vi "Predet_Inject.vi"   [LabVIEW 2017]
uses:
  <vilib>/DAQmx/write.llb/DAQmx Write (Digital 1D Wfm NChan NSamp).vi
  <vilib>/DAQmx/create/channels.llb/DAQmx Create Channel (DO-Digital Output).vi
  <vilib>/DAQmx/configure/timing.llb/DAQmx Timing (Sample Clock).vi
  <vilib>/Waveform/DWDTOps.llb/DWDT Uncompress Digital.vi
  <vilib>/DAQmx/miscellaneous.llb/DAQmx Fill In Error Info.vi
  <resource>/objmgr/daqmx.rc
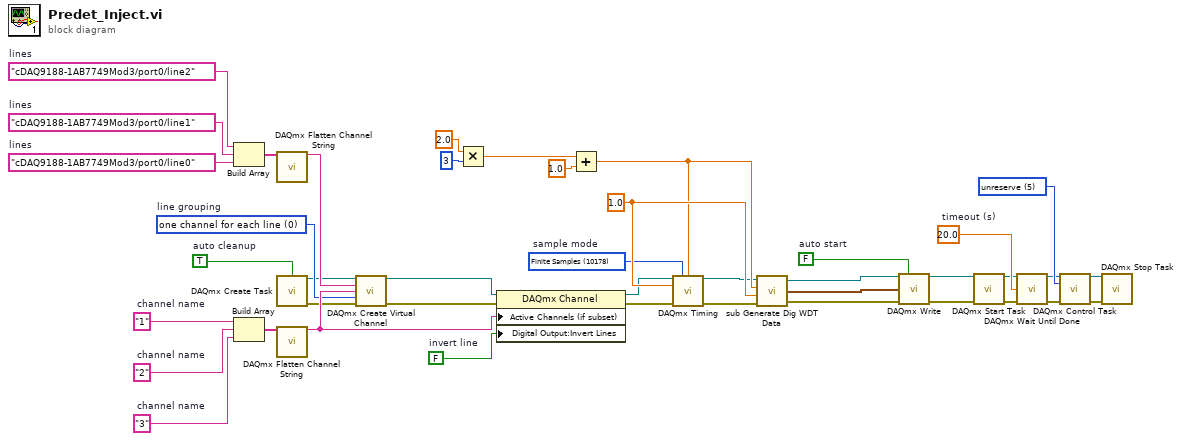
[diagram p0: block diagram]
diagram:
  w42 = 1.0 ("Predet Freq (Hz)")
  w40 = 5 items=["verify"=2, "reserve"=4, "commit"=3, "unreserve"=5, "abort"=6] ("action")
  w31 = "3"  # channel name
  w30 = "2"  # channel name
  w24 = "cDAQ9188-1AB7749Mod3/port0/line2"  # lines
  w25 = "cDAQ9188-1AB7749Mod3/port0/line1"  # lines
  w17 = 10178 items=["Finite Samples"=10178, "Continuous Samples"=10123, "Hardware Timed Single Point"=12522]  # sample mode
  w15 = FALSE  # invert line
  w11 = 0 items=["one channel for each line", "one channel for all lines"]  # line grouping
  w29 = "1"  # channel name
  w27 = "cDAQ9188-1AB7749Mod3/port0/line0"  # lines
  w9 = TRUE  # auto cleanup
  w7 = 20.0  # timeout (s)
  w1 = FALSE  # auto start
  n1 = Build Array(w24, w25, w27) -> (w26:string[])
  n2 = Build Array(w29, w30, w31) -> (w32:string[])
  n3 = call <vilib>:"DAQmx Flatten Channel String.vi"("names in"=w26) -> ("names out"=w28:string)  [unwired: 13 in, 1 out]
  n4 = call <vilib>:"DAQmx Create Task.vi"("auto cleanup"=w9) -> ("task out"=w10:refnum<k21>, "error out"=w8:errorcluster)  [unwired: 4 in, 9 out]
  n5 = call <vilib>:"DAQmx Flatten Channel String.vi"("names in"=w32) -> ("names out"=w33:string)  [unwired: 13 in, 1 out]
  n6 = call-poly <vilib>:"DAQmx Create Virtual Channel.vi"("task in"=w10, "lines"=w28, "name to assign"=w33, "line grouping"=w11, "error in"=w8) -> ("task out"=w12:refnum<k21>, "error out"=w13:errorcluster)  [unwired: 9 out]
  n7 = Multiply(x=2.0, y=3) -> (x*y=w21:dbl)
  n8 = property class="DAQmx Channel"(reference=w12, error in=w13, "Active Channels (if subset)"=w33, "Digital Output:Invert Lines"=w15) -> (reference out=w16:refnum<k21>, error out=w14:errorcluster)
  n9 = Add(x=w21, y=1.0) -> (x+y=w23:dbl)
  n10 = call-poly <vilib>:"DAQmx Timing.vi"("task/channels in"=w16, "sample mode"=w17, "samples per channel"=w23, "rate"=w42, "error in"=w14) -> ("task out"=w18:refnum<k21>, "error out"=w19:errorcluster)  [unwired: 2 in, 7 out]
  n11 = call <vilib>:"sub Generate Dig WDT Data.vi"("task in"=w18, "number of samples"=w23, "update rate"=w42, "error in"=w19) -> ("task out"=w3:refnum<k21>, "data"=w6:digitalwaveform[], "error out"=w2:errorcluster)  [unwired: 1 out]
  n12 = call-poly <vilib>:"DAQmx Write.vi"("task/channels in"=w3, "auto start"=w1, "data"=w6, "error in"=w2) -> ("task out"=w35:refnum<k21>, "error out"=w34:errorcluster)  [unwired: 10 out]
  n13 = call <vilib>:"DAQmx Start Task.vi"("task/channels in"=w35, "error in"=w34) -> ("task out"=w4:refnum<k21>, "error out"=w5:errorcluster)  [unwired: 12 out]
  n14 = call <vilib>:"DAQmx Wait Until Done.vi"("task/channels in"=w4, "timeout (sec)"=w7, "error in"=w5) -> ("task out"=w36:refnum<k21>, "error out"=w39:errorcluster)  [unwired: 11 out]
  n15 = call <vilib>:"DAQmx Control Task.vi"("task/channels in"=w36, "action"=w40, "error in"=w39) -> ("task out"=w37:refnum<k21>, "error out"=w38:errorcluster)  [unwired: 11 in]
  n16 = call <vilib>:"DAQmx Stop Task.vi"("task/channels in"=w37, "error in"=w38) -> ()  [unwired: 12 in, 2 out]
